vi "Read Mutation Rate.vi"(8 "error in (no error)":errorcluster, 11 "GA Core in":refnum<class "GA Core.lvclass">) -> (0 "error out":errorcluster, 2 "Mutation Rate":dbl, 3 "GA Core out":refnum<class "GA Core.lvclass">)   [LabVIEW 2016, in "GA Core.lvclass"]
uses:
  GA Core.lvclass
  GA Core.lvclass/GA Core.ctl
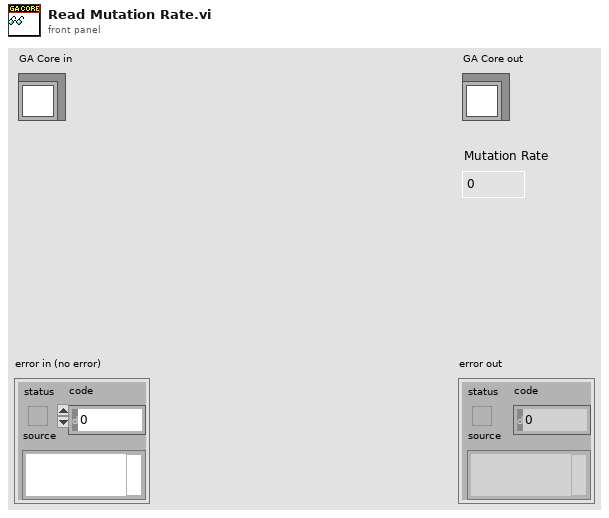
[diagram p1: front panel]
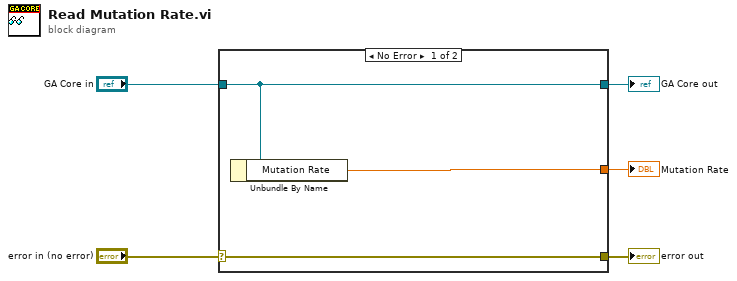
[diagram p0: block diagram]
diagram:
  n1 = case shown="No Error" "error in (no error)" {
    selector: "error in (no error)" -> [w8 w9]
    tunnel: [w8 w9] -> w4
    tunnel: [w7 w10] -> w2
    tunnel: "GA Core in" -> [w7 w10]
    tunnel: [w6 _] -> w1
    frame No Error {
      n2 = Unbundle By Name(w7) -> ("Mutation Rate"=w6:dbl)
    }
    frame Error {
    }
  }
  "error out" <- w4
  "GA Core out" <- w2
  "Mutation Rate" <- w1
